vi "display Aperture status.vi"(8 "error in":errorcluster={"status"=FALSE, "code"=-1950679034, "source"="Shared Variable in Large VAC READBACKS.vi<APPEND>\nThis error or warning occurred while reading the following Shared Variable:\n\\\\My Computer\\lowendshmc\\digital outputs\n\\\\192.168.1.200\\lowendshmc\\digital outputs"}, 9 "Aperture Status":T1, 10 "Actuator":bool=TRUE, 11 "Aperture display Refnum":refnum<vi>) -> (0 "error out":errorcluster={"status"=FALSE, "code"=-1950679034, "source"="Shared Variable in Large VAC READBACKS.vi<APPEND>\nThis error or warning occurred while reading the following Shared Variable:\n\\\\My Computer\\lowendshmc\\digital outputs\n\\\\192.168.1.200\\lowendshmc\\digital outputs"})   [LabVIEW 2016]
doc: "controls the display of if a cup or apt. is in the beamline"
uses:
  Controls/Aperture states.ctl
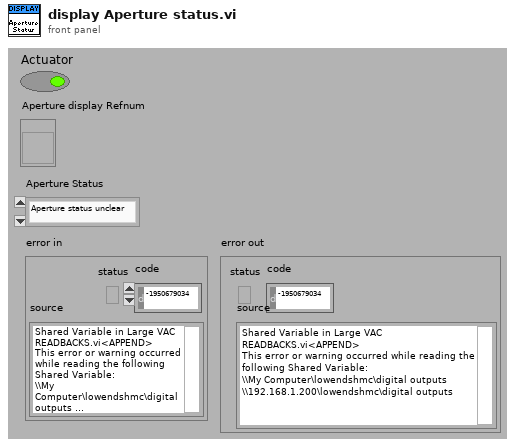
[diagram p1: front panel]
types:
  T1 = typedef "Aperture states.ctl" = enum16{"Aperture status unclear", "Aperture in", "Aperture out"}
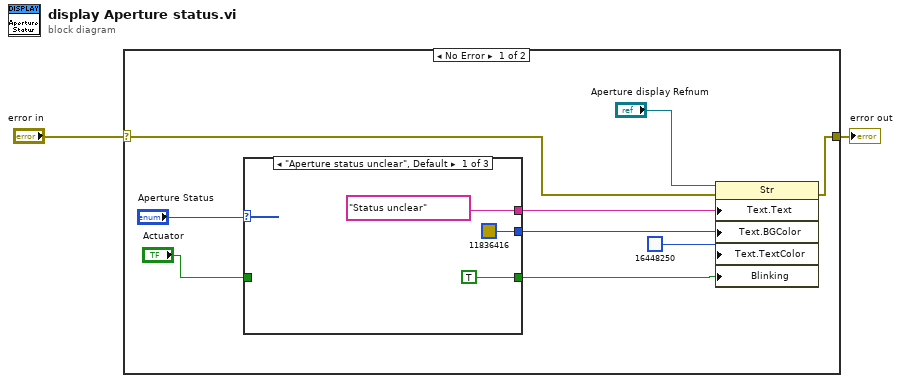
[diagram p0: block diagram]
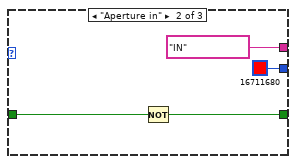
[diagram p2: hidden frame]
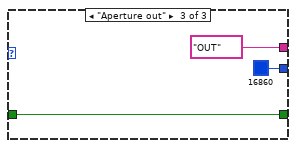
[diagram p3: hidden frame]
diagram:
  n1 = case shown="No Error" "error in" {
    selector: "error in" -> [w6 w22]
    tunnel: [w7 w22] -> w2
    frame No Error {
      n2 = case shown="\"Aperture status unclear\", Default" "Aperture Status" {
        tunnel: ["Status unclear" ("Text.Text") "IN" ("Text.Text") "OUT" ("Text.Text")] -> w9
        tunnel: [u32 11836416 u32 16711680 u32 16860] -> w10
        tunnel: [TRUE w15 w19] -> w5
        tunnel: "Actuator" -> [_ w16 w19]
        frame "Aperture status unclear", Default {
        }
        frame "Aperture in" {
          n3 = Not(x=w16) -> (.not. x?=w15:bool)
        }
        frame "Aperture out" {
        }
      }
      n4 = property on="Property Node" class="Str"(reference="Aperture display Refnum", error in=w6, "Text.Text"=w9, "Text.BGColor"=w10, "Text.TextColor"=u32 16448250, "Blinking"=w5) -> (error out=w7:errorcluster)  [unwired: 1 out]
    }
    frame Error {
    }
  }
  "error out" <- w2
